vi "array - rotate - row.vi"(6 "rotate row":i32, 11 "input matrix":T1) -> (3 "output matrix":T1)   [LabVIEW 2018]
uses:
  <vilib>/Analysis/Matrix/Datatypes/ComplexMatrix.ctl
  <vilib>/Analysis/Matrix/NI_Matrix.lvlib
panel:
  out "x-y*floor(x/y)":i32
  in  "dim":i32
  in  "rotate column":i32
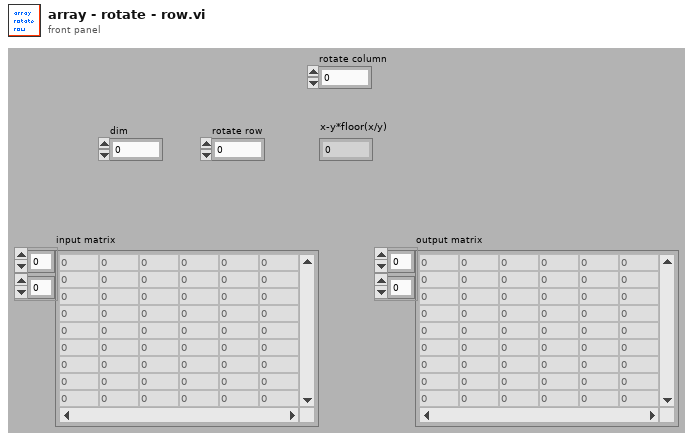
[diagram p1: front panel]
types:
  T1 = typedef "NI_Matrix.lvlib/ComplexMatrix.ctl" = cdb[][]
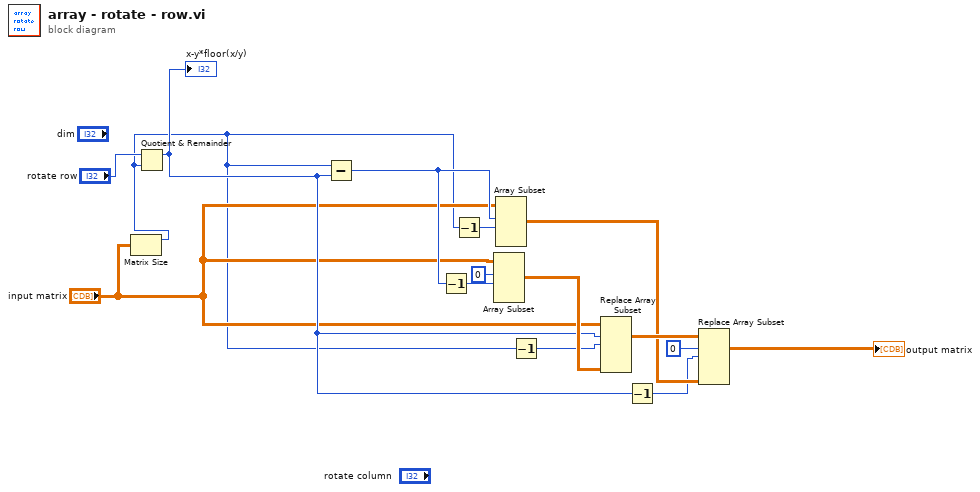
[diagram p0: block diagram]
diagram:
  n1 = Matrix Size(0:"input matrix") -> (1:w1:i32)  [unwired: 1 out]
  n2 = Quotient & Remainder(x="rotate row", y=w1) -> (x-y*floor(x/y)=w3:i32)  [unwired: 1 out]
  "x-y*floor(x/y)" <- w3
  n3 = Subtract(x=w1, y=w3) -> (x-y=w10:i32)
  n4 = Decrement(x=w10) -> (x-1=w9:i32)
  n5 = Decrement(x=w1) -> (x-1=w6:i32)
  n6 = Array Subset(array="input matrix", index (row)=0 ("row 1"), length (row)=w9) -> (w14:T1)  [unwired: 2 in]
  n7 = Array Subset(array="input matrix", index (row)=w10, length (row)=w6) -> (w8:T1)  [unwired: 2 in]
  n8 = Decrement(x=w1) -> (x-1=w7:i32)
  n9 = Replace Array Subset(array="input matrix", new element=w14, index (dim 0)=w3, index (dim 1)=w7) -> (w13:T1)  [unwired: 2 in]
  n10 = Decrement(x=w3) -> (x-1=w5:i32)
  n11 = Replace Array Subset(array=w13, new element=w8, index (dim 0)=0 ("row 1"), index (dim 1)=w5) -> (→"output matrix":T1)  [unwired: 2 in]
